vi "Send Schedules to Monkeys.vi"(8 "error in (no error)":errorcluster, 9 "Schedules":refnum<class "Schedule.lvclass">[](array[class]), 10 "Sync. Mask":T1[](array[typedef]), 11 "Tamer in":refnum<class "Tamer.lvclass">) -> (0 "error out":errorcluster, 3 "Tamer out":refnum<class "Tamer.lvclass">)   [LabVIEW 2020, in "TALOS.lvlib" / "Tamer.lvlib" / "Tamer.lvclass"]
uses:
  Tamer.lvclass
  Run Utilities/TypeDefs/Synchronize FPGA Cluster.ctl
  Run Utilities/Schedule/Schedule.lvclass
  C:/LabVIEW Code/TALOS/talos/Ancestor/Ancestor/Ancestor.lvclass
  C:/LabVIEW Code/TALOS/talos/Father of all uServices/Father of all uServices/Father of all uServices.lvclass
  Guardian/Guardian/Requests.ctl
  Run Utilities/TypeDefs/Messages/Schedule Message.ctl
  Run Utilities/TypeDefs/DAQ Control.ctl
  Run Utilities/TypeDefs/Monkey Status.ctl
  Ancestor/Ancestor/Ancestor.lvclass/Ancestor.ctl
  Guardian/Guardian Messages/Message to uService Msg/Message to uService Msg.lvclass/Message to uService Msg.ctl
  Guardian/Guardian Messages/Requests from uServices Msg/Requests from uServices Msg.lvclass/Requests from uServices Msg.ctl
  Ancestor/Ancestor/Read ID.vi
  Guardian/Guardian Messages/Message to uService Msg/Send Message to uService.vi
  Support VIs/Substitute Error.vi
  Guardian/Guardian Messages/Requests from uServices Msg/Send Requests from uServices.vi
  Support VIs/Generate Error.vi
  FGV/Error Memory/Get Error Description.vi
  Support VIs/Get PC name.vi
  Support VIs/Get Class Name.vi
  <vilib>/Utility/error.llb/Clear Errors.vi
  FGV/Error Memory/Error Memory Core.vi
  <vilib>/AdvancedString/Delimited String to 1D String Array.vi
  Support VIs/Circus Root Path.vi
  FGV/Error Memory/Error Crt Lvl checker.vi
  FGV/Error Memory/Error Memory Core.vi/40c8088d-b597-4017-91af-faa98e00292e.vi
  FGV/Error Memory/Error Memory Core.vi/d4a3ab98-063c-4e44-b43d-fbdcfe6c2be2.vi
  Father of all uServices/Father of all uServices/Father of all uServices.lvclass
  C:/LabVIEW Code/TALOS/builds/Actor Framework PPL/Actor Framework.lvlibp/1abvi3w/vi.lib/ActorFramework/Actor/Actor.lvclass
  builds/Actor Framework PPL/Actor Framework.lvlibp/1abvi3w/vi.lib/ActorFramework/Actor/Read Caller Enqueuer.vi
  builds/Actor Framework PPL/Actor Framework.lvlibp/1abvi3w/vi.lib/ActorFramework/Message Enqueuer/Enqueue.vi
  Support VIs/Global Memory.vi
  <vilib>/Utility/LVClass/Get LV Class Name.vi
  Support VIs/Is in Packed Library.vi
  Support VIs/TALOS Root path.vi
  Support VIs/Read CSV worksheet.vi
  Support VIs/Global Constants.vi
  <vilib>/Utility/error.llb/General Error Handler.vi
  Support VIs/Error Log.vi
  Guardian/Guardian Messages/Message to uService Msg/Message to uService Msg.lvclass
  Ancestor/Ancestor/Ancestor.lvclass
  <vilib>/Comparison/Equal/Equal Functor/Equal Functor.lvclass
  Guardian/Guardian Messages/Requests from uServices Msg/Requests from uServices Msg.lvclass
  Guardian/Guardian/Guardian.lvclass
  Run Utilities/Run Utilities.lvlib
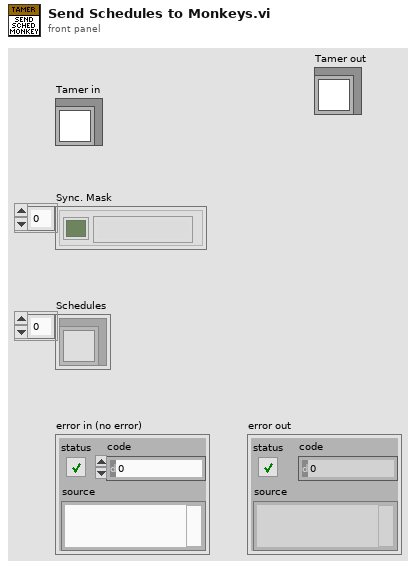
[diagram p1: front panel]
types:
  T1 = typedef "TALOS.lvlib/Run Utilities.lvlib/Synchronize FPGA Cluster.ctl" = cluster{"Status":bool, "FPGA Name":string}
  T2 = typedef "TALOS.lvlib/Guardian.lvlib/Guardian.lvclass/Requests.ctl" = enum16{"Ready to Launch", "Start RUN", "Stop RUN", "Update DAQ Params", "Update Error Listbox", "Update Run Status", "Update Kasli Log", "Run Stopped with Errors", "Switch uS View"}
  T3 = typedef "TALOS.lvlib/Run Utilities.lvlib/Monkey Status.ctl" = enum16{"Init", "Paused", "Ongoing", "Stopped", "Finished (no errors)", "Finished (with errors)"}
  T4 = typedef "TALOS.lvlib/Run Utilities.lvlib/Schedule Message.ctl" = cluster{"uS Name":string, "Synchronised":bool, "DAQ Control":T5, "Schedule":refnum<class "Schedule.lvclass">}
  T5 = typedef "TALOS.lvlib/Run Utilities.lvlib/DAQ Control.ctl" = enum16{"On", "Off", "External"}
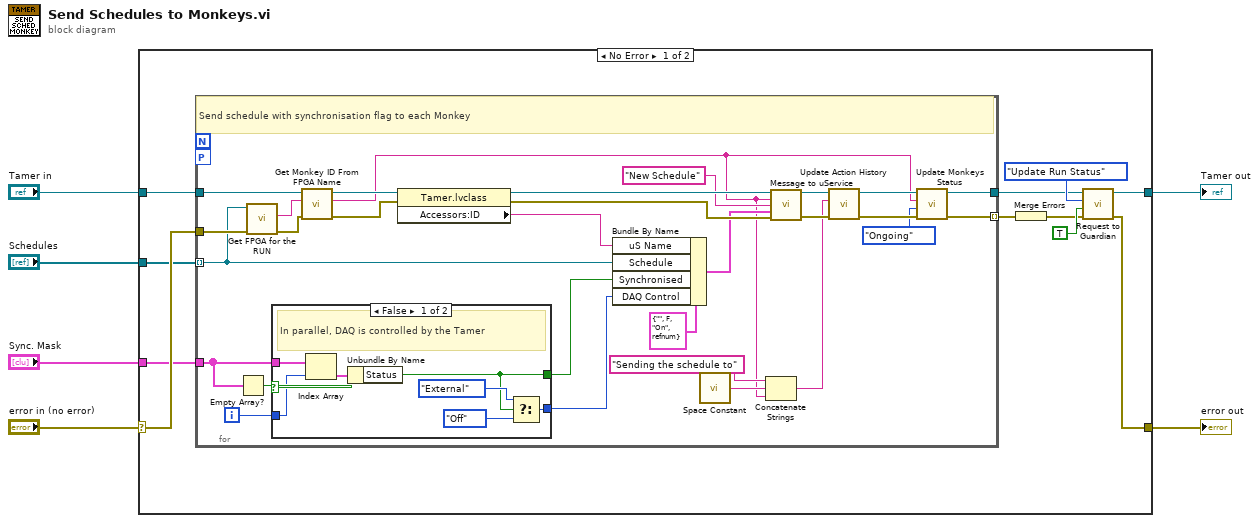
[diagram p0: block diagram]
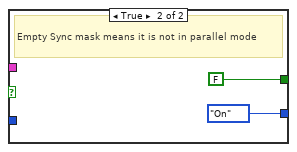
[diagram p2: hidden frame]
diagram:
  n1 = case shown="No Error" "error in (no error)" {
    selector: "error in (no error)" -> [w17 w57]
    tunnel: "Sync. Mask" -> [w16 _]
    tunnel: "Schedules" -> [w15 _]
    tunnel: "Tamer in" -> [w14 w56]
    tunnel: [w10 w57] -> w2
    tunnel: [w9 w56] -> w1
    frame No Error {
      n2 = for {
        tunnel: w14 -> [w31]
        tunnel: w15 -> [w18] mode=indexing
        tunnel: [w21] -> w8 mode=indexing
        tunnel: w16 -> [w39]
        tunnel: [w20] -> w11
        tunnel: w17 -> [w32]
        workers-P: _ -> [_]
        i -> [w40]
        # "Send schedule with synchronisation flag to each Monkey"
        n3 = Empty Array?(array=w39) -> (empty?=w41:bool)
        n4 = call-dynamic "Get FPGA for the RUN.vi"("error in (no error)"=w32, "Schedule in"=w18) -> ("error out"=w28:errorcluster, "FPGA Name"=w29:string)  [unwired: 7 in, 1 out]
        n5 = case shown="False" w41 {
          tunnel: [w47 FALSE] -> w23
          tunnel: w40 -> [w52 _]
          tunnel: w39 -> [w53 _]
          tunnel: [w50 DAQ_Control."On" ("DAQ Control")] -> w26
          frame False {
            # "In parallel, DAQ is controlled by the Tamer"
            n6 = Index Array(array=w53, index=w52) -> (element=w51:T1)
            n7 = Unbundle By Name(w51) -> ("Status"=w47:bool)
            n8 = Select(t=DAQ_Control."External" ("DAQ Control"), s=w47, f=DAQ_Control."Off") -> (s? t:f=w50:T5)
          }
          frame True {
            # "Empty Sync mask means it is not in parallel mode"
          }
        }
        n9 = call-dynamic "Get Monkey ID From FPGA Name.vi"("error in (no error)"=w28, "FPGA Name"=w29, "Tamer in"=w31) -> ("error out"=w27:errorcluster, "Monkey ID"=w22:string, "Tamer out"=w30:refnum<class "Tamer.lvclass">)  [unwired: 6 in]
        n10 = property class="Tamer.lvclass"(reference=w30, error in=w27) -> (reference out=w43:refnum<class "Tamer.lvclass">, error out=w46:errorcluster, "Accessors:ID"=w42:string)
        n11 = Bundle By Name(cluster=T4 {"uS Name"="", "Synchronised"=FALSE, "DAQ Control"=enum."On", "Schedule"=refnum} ("Monkey Schedule Message"), "uS Name"=w42, "Schedule"=w18, "Synchronised"=w23, "DAQ Control"=w26) -> (w45:T4)
        n12 = call <vilib>:"Space Constant.vi"() -> ("String"=w34:string)
        n13 = Concatenate Strings("Sending the schedule to" ("string"), w34, w22) -> (w36:string)
        n14 = call "Message to uService.vi"("Father of all uServices in"=w43, "uService ID"=w22, "Message"="New Schedule", "Data"=w45, "error in (no error)"=w46) -> ("Father of all uServices out"=w38:refnum<class "Tamer.lvclass">, "error out"=w37:errorcluster)  [unwired: 9 in]
        n15 = call-dynamic "Update Action History.vi"("error in (no error)"=w37, "Action"=w36, "Tamer in"=w38) -> ("error out"=w24:errorcluster, "Tamer out"=w25:refnum<class "Tamer.lvclass">)  [unwired: 7 in]
        n16 = call-dynamic "Update Monkeys Status.vi"("error in (no error)"=w24, "Status"=Monkey_Status."Ongoing", "Monkey ID"=w22, "Tamer in"=w25) -> ("error out"=w21:errorcluster, "Tamer out"=w20:refnum<class "Tamer.lvclass">)  [unwired: 6 in]
      }
      n17 = Merge Errors(w8) -> (w7:errorcluster)
      n18 = call "Request to Guardian.vi"("error in (no error)"=w7, "Data"=TRUE, "Requests"=Requests."Update Run Status", "Father of all uServices in"=w11) -> ("error out"=w10:errorcluster, "Father of all uServices out"=w9:refnum<class "Tamer.lvclass">)  [unwired: 6 in]
    }
    frame Error {
    }
  }
  "error out" <- w2
  "Tamer out" <- w1
